vi "Transfer.Get Intermediate Buffer.vi"(11 "Transfer in":refnum<class "Transfer.lvclass">) -> (2 "DBL Buffer":refnum<class "DBL Pointer.lvclass">, 3 "Transfer out":refnum<class "Transfer.lvclass">)   [LabVIEW 2017, in "DSF.Engine.lvlib" / "Transfer.lvclass"]
uses:
  Transfer.lvclass
  Pointer/DBL Pointer.lvclass
  Transfer.lvclass/Transfer.ctl
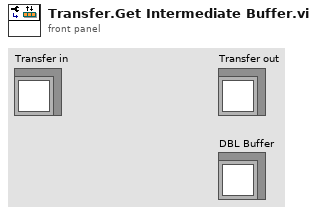
[diagram p1: front panel]
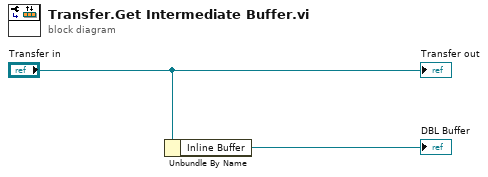
[diagram p0: block diagram]
diagram:
  n1 = Unbundle By Name("Transfer in") -> ("Inline Buffer"=→"DBL Buffer":refnum<class "DBL Pointer.lvclass">)
  "Transfer out" <- "Transfer in"
